vi "CRYGet Number to Window.vi"(4 "TSR Window Name":string, 5 "Weighting Name":string) -> (1 "TSR window":u16, 2 "Weighting":u16)   [LabVIEW 2013]
uses:
  Typedef Control/CRYWeigth Window.ctl
  Typedef Control/CRYTSR Window.ctl
panel:
  in  "TSR Window Type":T1 items=["None", "Cosine Tapered", "Half-Cosine Tapered", "Exponential", "Adrienne", "Half-Hanning", "Half-BH4"]
  in  "Weighting":T2 items=["None"=0, "Hanning"=1, "4 Term B-Harris"=7, "7 Term B-Harris"=8, "Flat Top"=6]
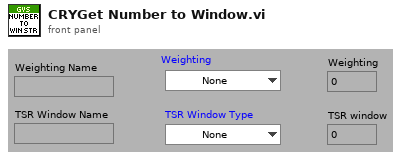
[diagram p1: front panel]
types:
  T1 = typedef "CRYTSR Window.ctl" = u16
  T2 = typedef "CRYWeigth Window.ctl" = u16
  T3 = typedef "LVStringsAndValuesArrayTypeDef_U16.ctl" = cluster{"String":string, "Value":u16}[]
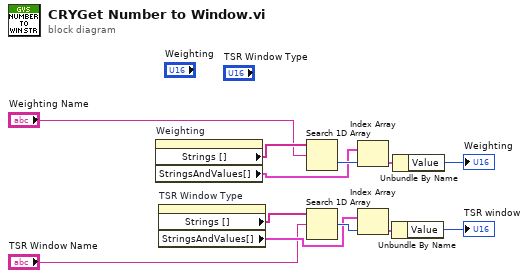
[diagram p0: block diagram]
diagram:
  n1 = property on="Weighting" class="Ring (strict)"() -> ("Strings []"=w5:string[], "StringsAndValues[]"=w7:T3)  [unwired: 2 in, 2 out]
  n2 = property on="TSR Window Type" class="Ring (strict)"() -> ("Strings []"=w6:string[], "StringsAndValues[]"=w9:T3)  [unwired: 2 in, 2 out]
  n3 = Search 1D Array(1D array=w5, element="Weighting Name") -> (index of element=w8:i32)  [unwired: 1 in]
  n4 = Search 1D Array(1D array=w6, element="TSR Window Name") -> (index of element=w10:i32)  [unwired: 1 in]
  n5 = Index Array(array=w7, index=w8) -> (element=w11:cluster{"String":string, "Value":u16})
  n6 = Index Array(array=w9, index=w10) -> (element=w12:cluster{"String":string, "Value":u16})
  n7 = Unbundle By Name(w12) -> ("Value"=→"TSR window":u16)
  n8 = Unbundle By Name(w11) -> ("Value"=→"Weighting":u16)
